vi "fpga_next_position_1ch_tip_guard.vi"(7 "speed":sgl, 8 "Tip guard position":sgl, 9 "tip guard?":bool, 10 "ready to move?":bool, 11 "target":sgl) -> (2 "move completed?":bool, 3 "output (out)":sgl)   [LabVIEW 2021]
doc: "This is a sub vi to calculate the next position.\n\nThis vi calculate a next position of single channel. The current position is stored in this vi."
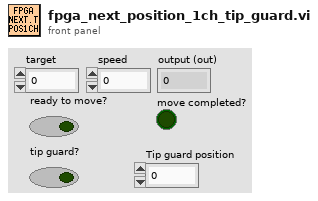
[diagram p1: front panel]
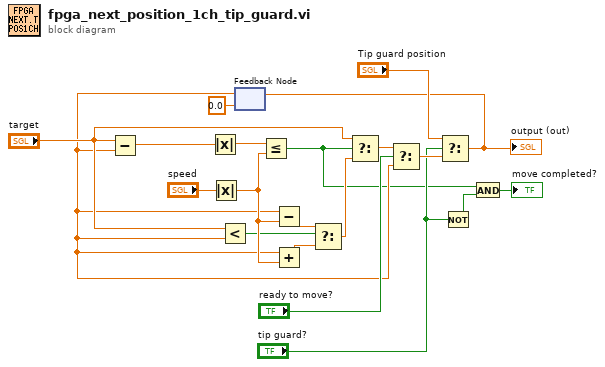
[diagram p0: block diagram]
diagram:
  n1 = Absolute Value(x="speed") -> (abs(x)=w19:sgl)
  n2 = feedback #1(sgl 0.0 ("target")) -> (w10:sgl)
  n3 = Subtract(x="target", y=w10) -> (x-y=w18:sgl)
  n4 = Absolute Value(x=w18) -> (abs(x)=w8:sgl)
  n5 = Less?(x="target", y=w10) -> (x < y?=w9:bool)
  n6 = Less Or Equal?(x=w8, y=w19) -> (x <= y?=w1:bool)
  n7 = Subtract(x=w10, y=w19) -> (x-y=w17:sgl)
  n8 = Add(x=w10, y=w19) -> (x+y=w16:sgl)
  n9 = Select(t=w17, s=w9, f=w16) -> (s? t:f=w15:sgl)
  n10 = Select(t="target", s=w1, f=w15) -> (s? t:f=w13:sgl)
  n11 = Select(t=w13, s="ready to move?", f=w10) -> (s? t:f=w6:sgl)
  n12 = Select(t="Tip guard position", s="tip guard?", f=w6) -> (s? t:f=w5:sgl)
  "output (out)" <- w5
  n13 = feedback-in #1(w5) -> ()
  n14 = Not(x="tip guard?") -> (.not. x?=w2:bool)
  n15 = And(x=w1, y=w2) -> (x .and. y?=→"move completed?":bool)
